vi "Get Variant.vi"(8 "error in (no error)":errorcluster, 11 "int32 in":refnum<class "packed.lvclass">) -> (0 "error out":errorcluster, 2 "Variant":variant, 3 "int32 out":refnum<class "packed.lvclass">)   [LabVIEW 2020, in "Protobuf RAW.lvlib" / "packed.lvclass"]
uses:
  packed.lvclass
  packed.lvclass/packed.ctl
  Scalar Encoder/Scalar Type.lvclass
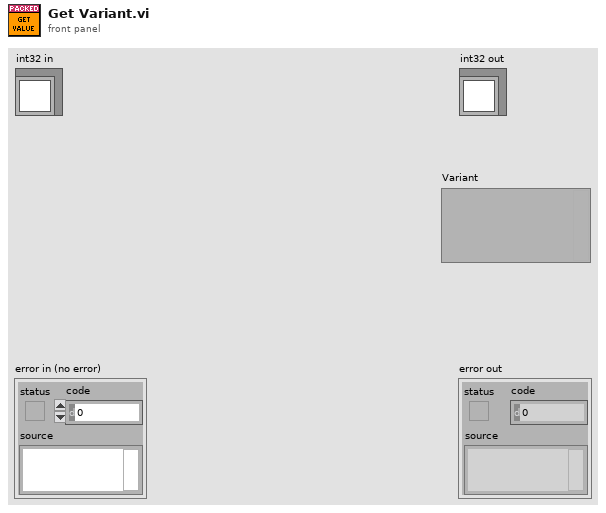
[diagram p1: front panel]
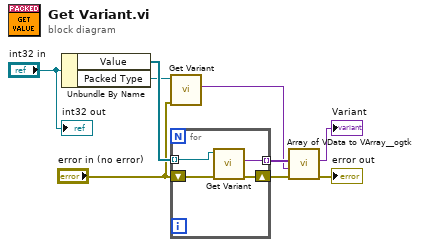
[diagram p0: block diagram]
diagram:
  n1 = Unbundle By Name("int32 in") -> ("Value"=w8:refnum<class "Scalar Type.lvclass">[], "Packed Type"=w5:refnum<class "Scalar Type.lvclass">)
  n2 = call-dynamic "Get Variant.vi"("error in (no error)"="error in (no error)", "Type Serializer in"=w5) -> ("Variant"=w3:variant)  [unwired: 7 in, 2 out]
  n3 = for {
    tunnel: w8 -> [w13] mode=indexing
    shift-right: [w11] -> w7
    shift-left: "error in (no error)" -> [w12]
    tunnel: [w10] -> w6 mode=indexing
    n4 = call-dynamic "Get Variant.vi"("error in (no error)"=w12, "Type Serializer in"=w13) -> ("error out"=w11:errorcluster, "Variant"=w10:variant)  [unwired: 7 in, 1 out]
  }
  n5 = call <userlib>:"Array of VData to VArray__ogtk.vi"("error in (no error)"=w7, "Element Type (when empty)"=w3, "1D Array of VData"=w6) -> ("error out"=→"error out":errorcluster, "VArray"=→"Variant":variant)  [unwired: 7 in]
  "int32 out" <- "int32 in"
